vi "Assert Stop.vi"(8 "error in (no error)":errorcluster, 11 "User Interface in":refnum<class "User Interface.lvclass">) -> (0 "error out":errorcluster, 3 "User Interface out":refnum<class "User Interface.lvclass">)   [LabVIEW 2017, in "DSF Core.lvlib" / "User Interface.lvclass"]
uses:
  User Interface.lvclass
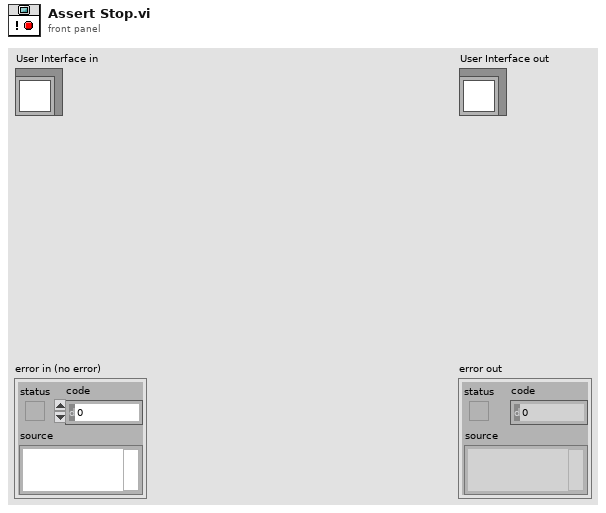
[diagram p1: front panel]
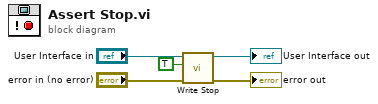
[diagram p0: block diagram]
diagram:
  n1 = call "Write Stop.vi"("error in (no error)"="error in (no error)", "stop"=TRUE, "User Interface in"="User Interface in") -> ("error out"=→"error out":errorcluster, "User Interface out"=→"User Interface out":refnum<class "User Interface.lvclass">)  [unwired: 7 in]
